vi "Trajectory_New.vi"(11 "TRAJ_STATES":T2[](array[typedef])) -> (3 "TRAJECTORY":T1 {"TotalTImeSecs" format="%20.3f"})   [LabVIEW 2019, in "Trajectory_Library.lvlib"]
doc: "Constructs a trajectory from a vector of states.\n\nRepresents a time-parameterized trajectory. The trajectory contains of various States that represent the pose, curvature, time elapsed, velocity, and acceleration at that point.\n\nParameters:\n - TrajStates - A vector of states.\n\nReturns:\n - Trajectory - Trajectory data structure"
uses:
  Trajectory_Library.lvlib
  TRAJ_STATE.ctl
  POSE2D.ctl
  TRANSLATION2D.ctl
  ROTATION2D.ctl
  TRAJECTORY.ctl
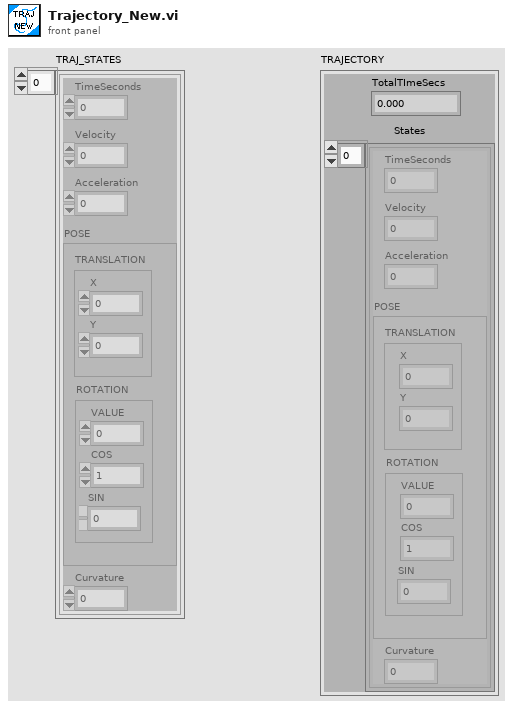
[diagram p1: front panel]
types:
  T1 = typedef "Trajectory_Library.lvlib/TRAJECTORY.ctl" = cluster{"TotalTImeSecs":dbl, "States":T2[]}
  T2 = typedef "Trajectory_Library.lvlib/TRAJ_STATE.ctl" = cluster{"TimeSeconds":dbl, "Velocity":dbl, "Acceleration":dbl, "POSE":T3, "Curvature":dbl}
  T3 = typedef "Trajectory_Library.lvlib/POSE2D.ctl" = cluster{"TRANSLATION":T4, "ROTATION":T5}
  T4 = typedef "Trajectory_Library.lvlib/TRANSLATION2D.ctl" = cluster{"X":dbl, "Y":dbl}
  T5 = typedef "Trajectory_Library.lvlib/ROTATION2D.ctl" = cluster{"VALUE":dbl, "COS":dbl, "SIN":dbl}
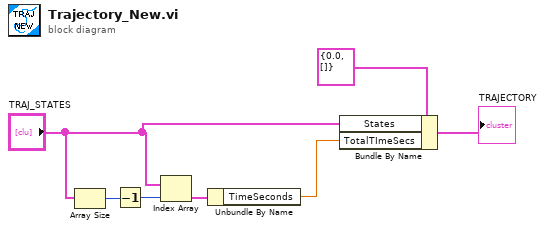
[diagram p0: block diagram]
diagram:
  n1 = Array Size(array="TRAJ_STATES") -> (size(s)=w5:i32)
  n2 = Decrement(x=w5) -> (x-1=w4:i32)
  n3 = Index Array(array="TRAJ_STATES", index=w4) -> (element=w3:T2)
  n4 = Unbundle By Name(w3) -> ("TimeSeconds"=w2:dbl)
  n5 = Bundle By Name(cluster=T1 {"TotalTImeSecs"=0.0, "States"=[]} ("TRAJECTORY"), "States"="TRAJ_STATES", "TotalTImeSecs"=w2) -> (→"TRAJECTORY":T1)
